vi "Transpose and Get Headers.vi"(11 "Channels per Device'":string[][](array[string])) -> (1 "Column Headers":string[](array[string]), 2 "Row Headers":string[](array[string]), 3 "Channels per Device":string[][](table))   [LabVIEW 2014]
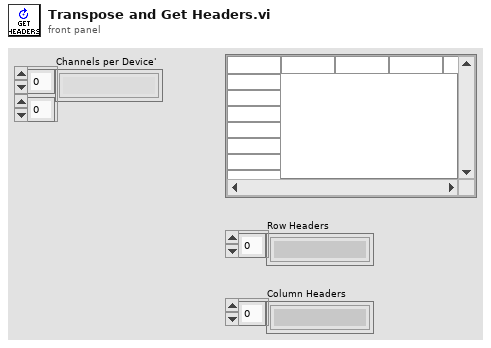
[diagram p1: front panel]
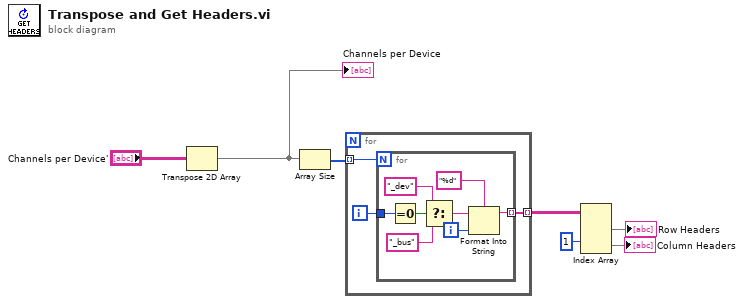
[diagram p0: block diagram]
diagram:
  n1 = Transpose 2D Array(2D array="Channels per Device'") -> (transposed array=w4:string[][])
  "Channels per Device" <- w4
  n2 = Array Size(array=w4) -> (size(s)=w7:i32[])
  n3 = for {
    tunnel: w7 -> [w10] mode=indexing
    tunnel: [w8] -> w6 mode=indexing
    i -> [w9]
    n4 = for {
      N: w10 -> [_]
      tunnel: w9 -> [w18]
      tunnel: [w11] -> w8 mode=indexing
      i -> [w12]
      n5 = Equal To 0?(x=w18) -> (x = 0?=w17:bool)
      n6 = Select(t="_dev", s=w17, f="_bus") -> (s? t:f=w14:string)
      n7 = Format Into String(format string="%d", initial string=w14, w12) -> (resulting string=w11:string)  [unwired: 1 in, 1 out]
    }
  }
  n8 = Index Array(array=w6, index (row) #2=1 ("index (row)")) -> (element #1=→"Row Headers":string[], element #2=→"Column Headers":string[])  [unwired: 3 in]
